vi "Create Cache.vi"() -> (3 "ConfigManager.Cache":refnum<class "ConfigManager.Cache.lvclass">)   [LabVIEW 2013, in "CfgManager.lvlib" / "ConfigManager.Cache.lvclass"]
uses:
  ConfigManager.Cache.lvclass
  ConfigManager.Cache.lvclass/ConfigManager.Cache.ctl
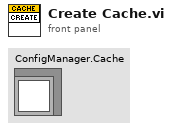
[diagram p1: front panel]
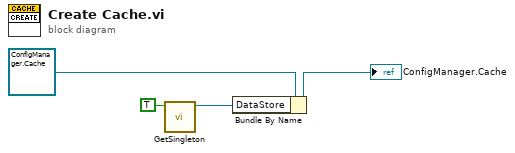
[diagram p0: block diagram]
diagram:
  n1 = call "GetSingleton.vi"("Creator (F)"=TRUE) -> ("DataStore"=w3:refnum<data-value>)  [unwired: 9 in, 1 out]
  n2 = Bundle By Name(cluster=refnum<class "ConfigManager.Cache.lvclass"> refnum ("SMOConfigManagerCollection.lvclass"), "DataStore"=w3) -> (→"ConfigManager.Cache":refnum<class "ConfigManager.Cache.lvclass">)
